vi "SetDisplayInput.vi"(8 "error in (no error)":errorcluster, 9 "Test":string, 10 "Wafer ID":string, 11 "EpiWrapper in":refnum<class "EpiWrapper.lvclass">) -> (0 "error out":errorcluster, 3 "EpiWrapper out":refnum<class "EpiWrapper.lvclass">)   [LabVIEW 2012, in "EpiWrapper.lvclass"]
uses:
  EpiWrapper.lvclass
  Controls/UserInput.ctl
  EpiWrapper.lvclass/EpiWrapper.ctl
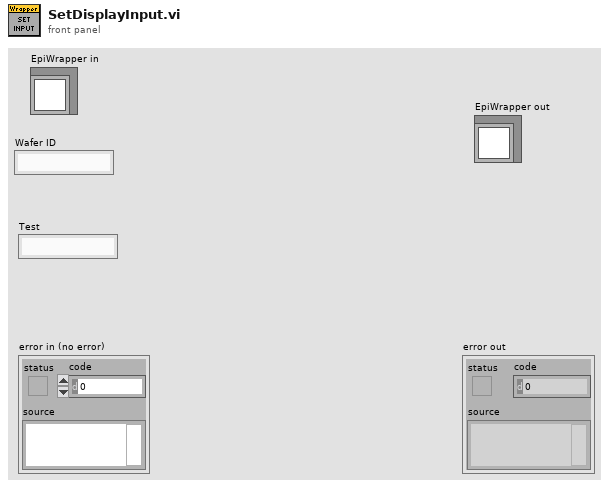
[diagram p1: front panel]
types:
  T1 = typedef "UserInput.ctl" = cluster{"Wafer ID":string, "Test":string, "New":bool, "Save":bool, "Load":bool, "Cancel":bool}
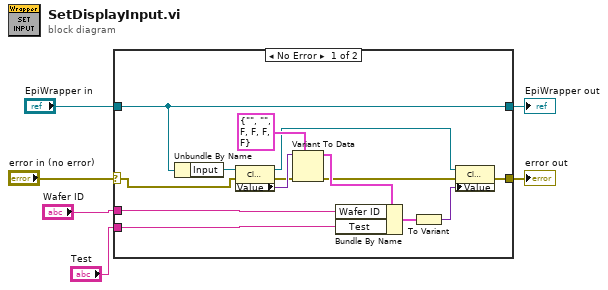
[diagram p0: block diagram]
diagram:
  n1 = case shown="No Error" "error in (no error)" {
    selector: "error in (no error)" -> [w7 w22]
    tunnel: [w9 w22] -> w5
    tunnel: [w8 w21] -> w3
    tunnel: "EpiWrapper in" -> [w8 w21]
    tunnel: "Wafer ID" -> [w16 _]
    tunnel: "Test" -> [w15 _]
    frame No Error {
      n2 = Unbundle By Name(w8) -> ("Input"=w17:refnum<vi>)
      n3 = property class="Clust"(reference=w17, error in=w7) -> (reference out=w13:refnum<vi>, error out=w19:errorcluster, "Value"=w20:variant)
      n4 = Variant To Data(error in=w19, type=T1 {"Wafer ID"="", "Test"="", "New"=FALSE, "Save"=FALSE, "Load"=FALSE, "Cancel"=FALSE} ("Cluster 2"), Variant=w20) -> (data=w14:T1, error out=w12:errorcluster)
      n5 = Bundle By Name(cluster=w14, "Wafer ID"=w16, "Test"=w15) -> (w10:T1)
      n6 = To Variant(anything=w10) -> (Variant=w11:variant)
      n7 = property class="Clust"(reference=w13, error in=w12, "Value"=w11) -> (error out=w9:errorcluster)  [unwired: 1 out]
    }
    frame Error {
    }
  }
  "error out" <- w5
  "EpiWrapper out" <- w3
